vi "Test D13 Toggle.vi"() -> ()   [LabVIEW 2014]
panel:
  out "Error Out":errorcluster
  in  "Error In":errorcluster
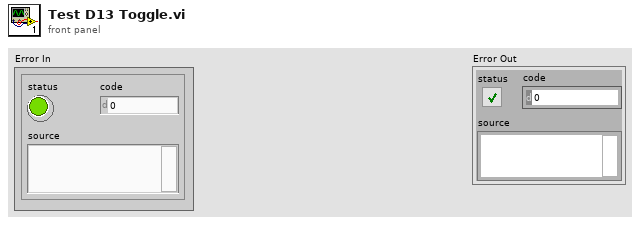
[diagram p1: front panel]
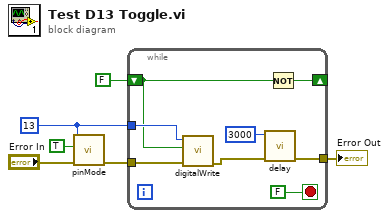
[diagram p0: block diagram]
diagram:
  w3 = 13 ("pin number")
  n1 = call <vilib>:"pinMode.vi"("Error In"="Error In", "output?"=TRUE, "pin number"=w3) -> ("Error Out"=w4:errorcluster)  [unwired: 8 in]
  n2 = while {
    tunnel: w4 -> [w14]
    tunnel: w3 -> [w13]
    shift-right: [w11] -> _
    shift-left: FALSE ("output?") -> [w12]
    tunnel: [w8] -> w1
    stop <- FALSE stop-if-true
    n3 = call <vilib>:"digitalWrite.vi"("Error In"=w14, "value"=w12, "pin number"=w13) -> ("Error Out"=w10:errorcluster)  [unwired: 8 in]
    n4 = call <vilib>:"delay.vi"("Error In"=w10, "time (ms)"=3000) -> ("Error Out"=w8:errorcluster)  [unwired: 9 in]
    n5 = Not(x=w12) -> (.not. x?=w11:bool)
  }
  "Error Out" <- w1
